vi "Update.vi"() -> ()   [LabVIEW 2018]
panel:
  out "standard error 3":string
  out "standard output 3":string
  out "name":string
  out "exists":bool
  out "is directory":bool
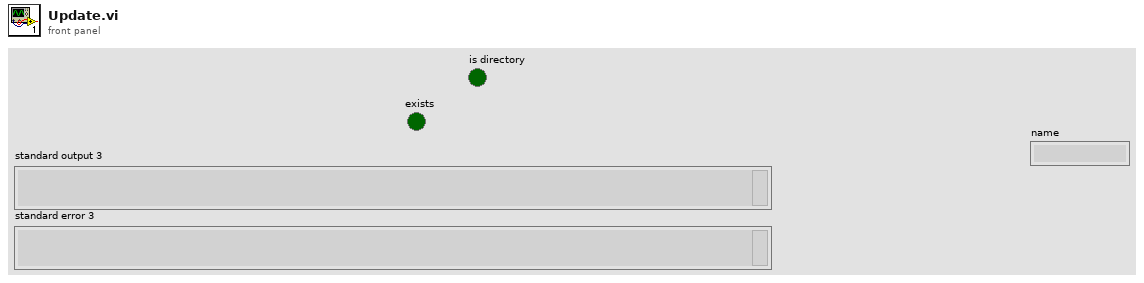
[diagram p1: front panel]
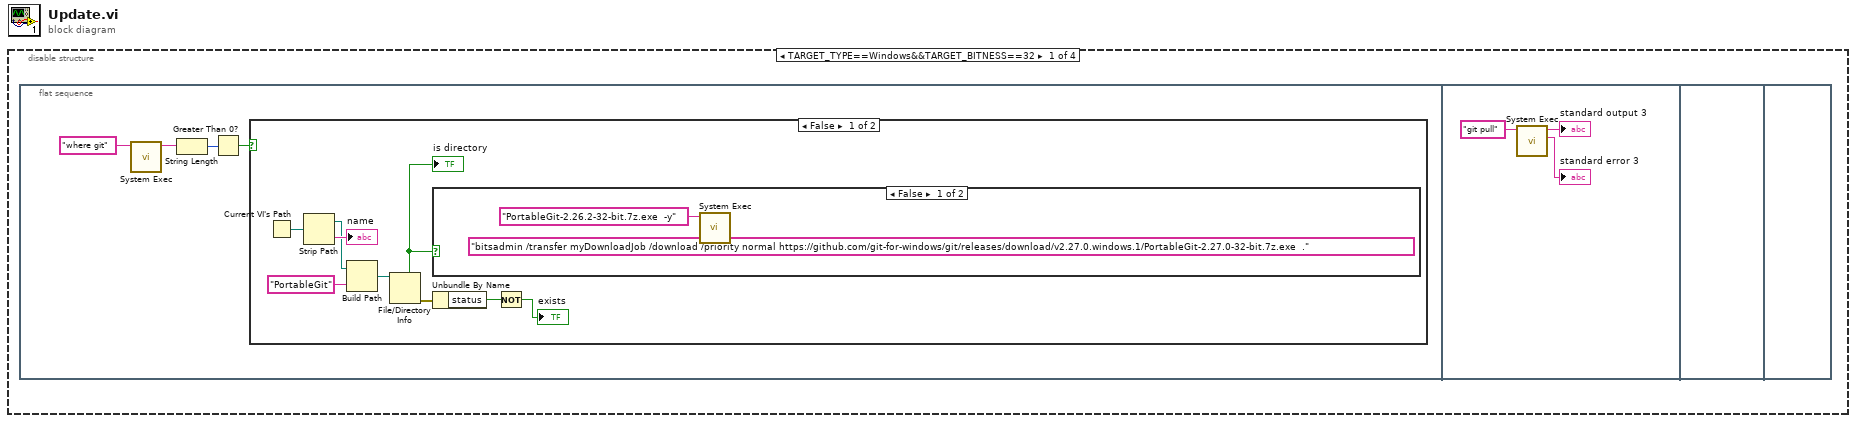
[diagram p0: block diagram]
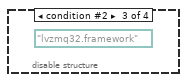
[diagram p5: hidden frame]
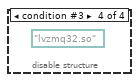
[diagram p6: hidden frame]
diagram:
  n1 = disable-structure shown="TARGET_TYPE==Windows&&TARGET_BITNESS==32" {
    frame condition #0 (active) {
      n2 = flat-sequence {
        frame #0 {
          n3 = call <vilib>:"System Exec.vi"("command line"="where git") -> ("standard output"=w3:string)  [unwired: 7 in, 3 out]
          n4 = String Length(string=w3) -> (length=w2:i32)
          n5 = Greater Than 0?(x=w2) -> (x > 0?=w1:bool)
          n6 = case shown="False" w1 {
            frame False {
              n7 = Current VI's Path() -> (path=w13:path)
              n8 = Strip Path(path=w13) -> (stripped path=w10:path, name=→"name":string)
              n9 = Build Path(base path=w10, name or relative path="PortableGit") -> (appended path=w7:path)
              n10 = File/Directory Info(path=w7) -> (directory=w6:bool, error out=w9:errorcluster)  [unwired: 1 in, 5 out]
              "is directory" <- w6
              n11 = case shown="False" w6 {
                frame False {
                  (unwired) "bitsadmin /transfer myDownloadJob /download /priority normal https://github.com/git-for-windows/git/releases/download/v2.27.0.windows.1/PortableGit-2.27.0-32-bit.7z.exe  ."
                  n12 = call <vilib>:"System Exec.vi"("command line"="PortableGit-2.26.2-32-bit.7z.exe  -y") -> ()  [unwired: 7 in, 4 out]
                }
                frame True {
                }
              }
              n13 = Unbundle By Name(w9) -> ("status"=w8:bool)
              n14 = Not(x=w8) -> (.not. x?=→"exists":bool)
            }
            frame True {
            }
          }
        }
        frame #1 {
          n15 = call <vilib>:"System Exec.vi"("command line"="git pull") -> ("standard error"=→"standard error 3":string, "standard output"=→"standard output 3":string)  [unwired: 7 in, 2 out]
        }
        frame #2 {
        }
        frame #3 {
        }
      }
    }
    frame condition #1 {
    }
    frame condition #2 {
      w18 = path "lvzmq32.framework" ("appended path")
    }
    frame condition #3 {
      w19 = path "lvzmq32.so" ("appended path")
    }
  }
